vi "Set Var.vi"(8 "error in (no error)":errorcluster caption="错误输入（无错误）", 10 "Var":variant, 11 "Contstant Base输入":refnum<class "Tag Data.lvclass">) -> (0 "error out":errorcluster caption="错误输出", 3 "Contstant Base输出":refnum<class "Tag Data.lvclass">)   [LabVIEW 2013, in "Tag Data.lvclass"]
uses:
  Tag Data.lvclass
  Tag Data.lvclass/Tag Data.ctl
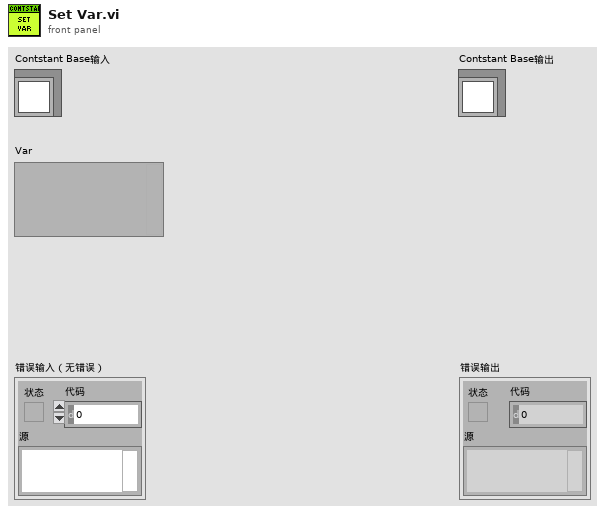
[diagram p1: front panel]
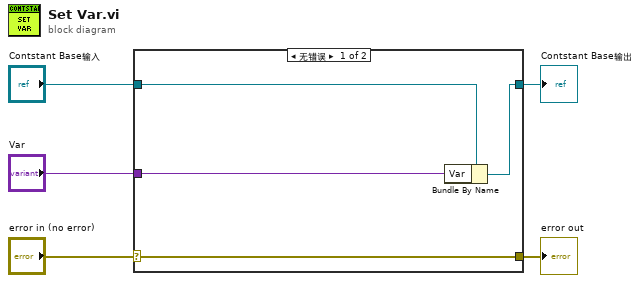
[diagram p0: block diagram]
diagram:
  n1 = case shown="无错误" "error in (no error)" {
    selector: "error in (no error)" -> [w9 w10]
    tunnel: [w9 w10] -> w4
    tunnel: [w7 w11] -> w2
    tunnel: "Contstant Base输入" -> [w8 w11]
    tunnel: "Var" -> [w6 _]
    frame No Error {
      n2 = Bundle By Name(cluster=w8, "Var"=w6) -> (w7:refnum<class "Tag Data.lvclass">)
    }
    frame Error {
    }
  }
  "error out" <- w4
  "Contstant Base输出" <- w2
